vi "ASCII2HEX.vi"(8 "String (Normal Display)":string) -> (0 "Result string (Hex Display)":string)   [LabVIEW 2011]
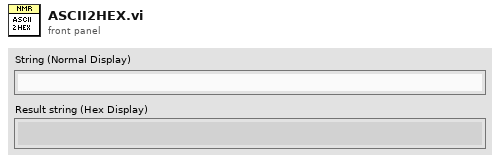
[diagram p1: front panel]
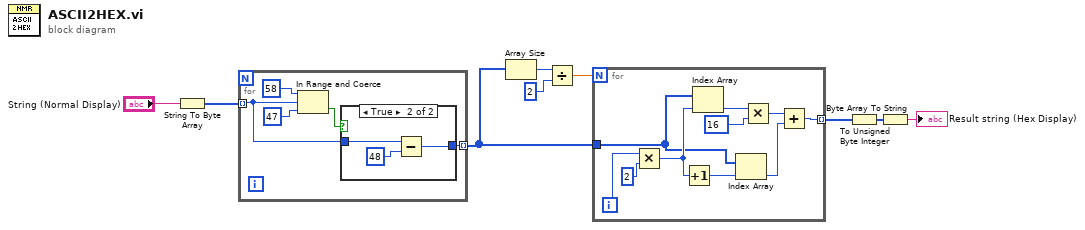
[diagram p0: block diagram]
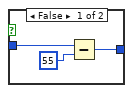
[diagram p2: hidden frame]
diagram:
  n1 = String To Byte Array(string="String (Normal Display)") -> (unsigned byte array=w8:u8[])
  n2 = for {
    tunnel: w8 -> [w11] mode=indexing
    tunnel: [w10] -> w4 mode=indexing
    n3 = In Range and Coerce(upper limit=u8 58 ("x"), x=w11, lower limit=u8 47) -> (In Range?=w12:bool)  [unwired: 1 out]
    n4 = case shown="True" w12 {
      tunnel: w11 -> [w16 w20]
      tunnel: [w15 w18] -> w10
      frame False {
        n5 = Subtract(x=w16, y=u8 55) -> (x-y=w15:u8)
      }
      frame True {
        n6 = Subtract(x=w20, y=u8 48) -> (x-y=w18:u8)
      }
    }
  }
  n7 = Array Size(array=w4) -> (size(s)=w7:i32)
  n8 = Divide(x=w7, y=2) -> (x/y=w5:dbl)
  n9 = for {
    N: w5 -> [_]
    tunnel: w4 -> [w23]
    tunnel: [w21] -> w3 mode=indexing
    i -> [w30]
    n10 = Multiply(x=w30, y=2) -> (x*y=w24:i32)
    n11 = Increment(x=w24) -> (x+1=w25:i32)
    n12 = Index Array(array=w23, index=w24) -> (element=w28:u8)
    n13 = Index Array(array=w23, index=w25) -> (element=w22:u8)
    n14 = Multiply(x=w28, y=16) -> (x*y=w26:i32)
    n15 = Add(x=w26, y=w22) -> (x+y=w21:i32)
  }
  n16 = To Unsigned Byte Integer(number=w3) -> (unsigned 8bit integer=w1:u8[])
  n17 = Byte Array To String(unsigned byte array=w1) -> (string=→"Result string (Hex Display)":string)
